vi "Connect.vi"(8 "error in (no error)":errorcluster, 10 "Connection String":string, 11 "dbcDotNet Type":refnum<class "ORM_DBC_dotNet.lvclass">) -> (0 "error out":errorcluster, 3 "dbcDotNet out":refnum<class "ORM_DBC_dotNet.lvclass">)   [LabVIEW 2020, in "ORM_DBC_dotNet.lvlib" / "ORM_DBC_dotNet.lvclass"]
uses:
  ORM_DBC_dotNet.lvclass
  <vilib>/Viviota/shared/ORM.lvlibp/ORM/DbConnection/DbConnection.lvclass
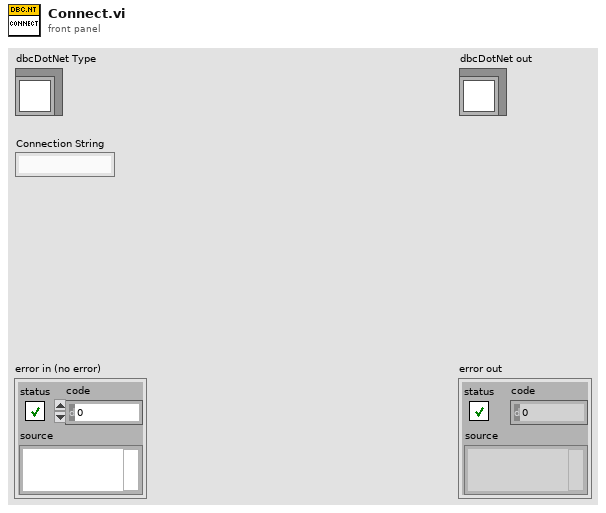
[diagram p1: front panel]
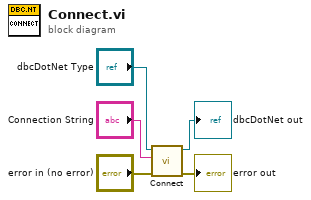
[diagram p0: block diagram]
diagram:
  n1 = call-parent "Connect.vi"("error in (no error)"="error in (no error)", "Connection String"="Connection String", "DbConnection Type"="dbcDotNet Type") -> ("error out"=→"error out":errorcluster, "DbConnection out"=→"dbcDotNet out":refnum<class "ORM_DBC_dotNet.lvclass">)  [unwired: 7 in]
